vi "ConstructPath.vi"(11 "Segments":string[](array[string])) -> (3 "path":string)   [LabVIEW 2013, in "openURI.lvlib"]
uses:
  openURI.lvlib
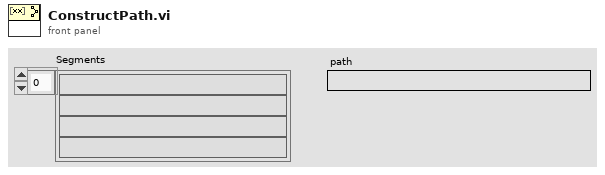
[diagram p1: front panel]
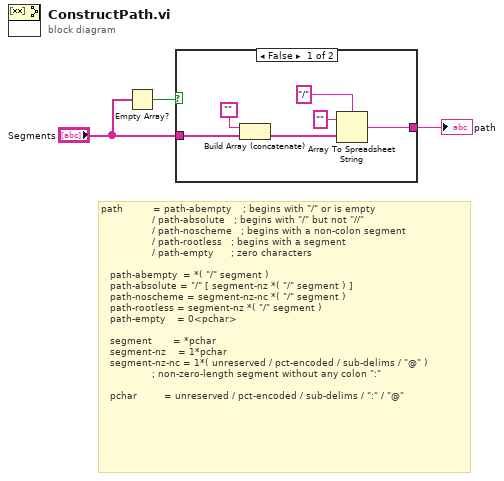
[diagram p0: block diagram]
diagram:
  # "path          = path-abempty    ; begins with \"/\" or is empty\n                 / path-absolute   ; begins with \"/\" but not \"//\"\n                 / path-noscheme   ; begins with a non-colon segment\n                 / path-rootless   ; begins with a segment\n                 / path-empty      ; zero characters\n\n   path-abempty  = *( \"/\" segment )\n   path-absolute = \"/\" [ segment-nz *( \"/\" segment ) ]\n   path-noscheme = segment-nz-nc *( \"/\" segment )\n   path-rootless = segment-nz *( \"/\" segment )\n   path-empty    = 0<pchar>\n\n   segment       = *pchar\n   segment-nz    = 1*pchar\n   segment-nz-nc = 1*( unreserved / pct-encoded / sub-delims / \"@\" )\n                 ; non-zero-length segment without any colon \":\"\n\n   pchar         = unreserved / pct-encoded / sub-delims / \":\" / \"@\""
  n1 = Empty Array?(array="Segments") -> (empty?=w3:bool)
  n2 = case shown="False" w3 {
    tunnel: "Segments" -> [w5 _]
    tunnel: [w7 _] -> w1
    frame False {
      n3 = Build Array (concatenate)("", w5) -> (w4:string[])
      n4 = Array To Spreadsheet String(delimiter (Tab)="/", array=w4, 3:"" ("format string")) -> (spreadsheet string=w7:string)
    }
    frame True {
    }
  }
  "path" <- w1
